vi "calculate_moving_average.vi"(6 "dimension size":i32, 7 "vertical? (N)":bool, 11 "array in":dbl[][](array[numeric])) -> (3 "array out":dbl[][](array[numeric]))   [LabVIEW 2010, in "AnalysisRaps2.lvclass"]
uses:
  AnalysisRaps2.lvclass
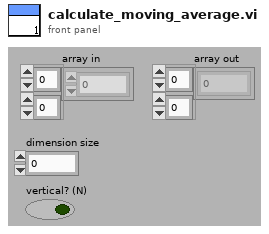
[diagram p1: front panel]
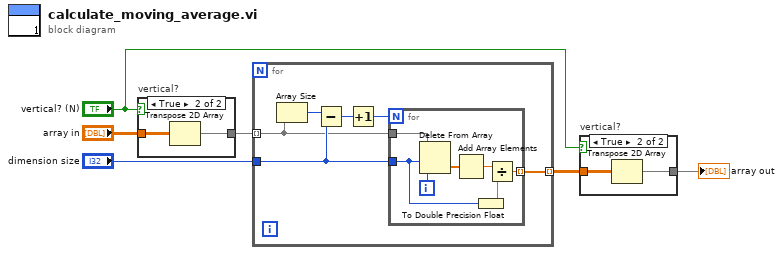
[diagram p0: block diagram]
diagram:
  n1 = case "vertical?" shown="True" "vertical? (N)" {
    tunnel: "array in" -> [w7 w9]
    tunnel: [w7 w8] -> w4
    frame False {
    }
    frame True {
      n2 = Transpose 2D Array(2D array=w9) -> (transposed array=w8:dbl[][])
    }
  }
  n3 = for {
    tunnel: "dimension size" -> [w15]
    tunnel: [w12] -> w3 mode=indexing
    tunnel: w4 -> [w10] mode=indexing
    n4 = Array Size(array=w10) -> (size(s)=w14:i32)
    n5 = Subtract(x=w14, y=w15) -> (x-y=w13:i32)
    n6 = Increment(x=w13) -> (x+1=w11:i32)
    n7 = for {
      N: w11 -> [_]
      tunnel: w10 -> [w22]
      tunnel: w15 -> [w20]
      tunnel: [w18] -> w12 mode=indexing
      i -> [w17]
      n8 = Delete From Array(array=w22, length=w20, index=w17) -> (deleted portion=w16:dbl[])  [unwired: 1 out]
      n9 = Add Array Elements(numeric array=w16) -> (sum=w21:dbl)
      n10 = To Double Precision Float(number=w20) -> (double precision float=w19:dbl)
      n11 = Divide(x=w21, y=w19) -> (x/y=w18:dbl)
    }
  }
  n12 = case "vertical?" shown="True" "vertical? (N)" {
    tunnel: w3 -> [w23 w25]
    tunnel: [w23 w24] -> w2
    frame False {
    }
    frame True {
      n13 = Transpose 2D Array(2D array=w25) -> (transposed array=w24:dbl[][])
    }
  }
  "array out" <- w2
